vi "GetTemperatureSD.vi"(4 "error in (no error)":errorcluster) -> (0 "error out":errorcluster, 1 "DLL error code":u32, 2 "status":T1, 3 "temperature":i32)   [LabVIEW 2015]
doc: "This function returns the temperature of the detector to the nearest degree. It also gives the status of cooling process.\n\n<B>Parameter:</B>\ntemperature - temperature of the detector\nstatus - status of cooling process\n\n<B>Error codes:</B>\nDRV_NOT_INITIALIZED - System not initialized.\nDRV_ACQUIRING - Acquisition in progress.\nDRV_ERROR_ACK - Unable to communicate with card.\nDRV_TEMP_OFF - Temperature is OFF.\nDRV_TEMP_STABILIZED - Temperature has stabilized at set point.\nDRV_TEMP_NOT_REACHED - Temperature has not reached set point."
uses:
  Error Code Enum typedef.ctl
  DLL/atmcd32d.dll
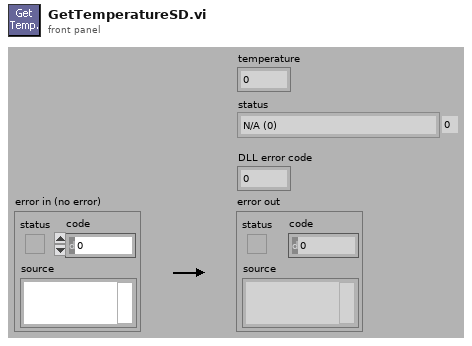
[diagram p1: front panel]
types:
  T1 = typedef "Error Code Enum typedef.ctl" = enum32{"N/A (0)", "DRV_ERROR_CODES", "DRV_SUCCESS", "DRV_VXDNOTINSTALLED", "DRV_ERROR_SCAN", "DRV_ERROR_CHECK_SUM", "DRV_ERROR_FILELOAD", "DRV_UNKNOWN_FUNC", "DRV_ERROR_VXD_INIT", "DRV_ERROR_ADDRESS", "DRV_ERROR_PAGELOCK", "DRV_ERROR_PAGEUNLOCK", "DRV_ERROR_BOARDTEST", "DRV_ERROR_ACK", "DRV_ERROR_UP_FIFO", "DRV_ERROR_PATTERN", "N/A (16)", "DRV_ACQUISITION_ERRORS", "DRV_ACQ_BUFFER", "DRV_ACQ_DOWNFIFO_FULL", "DRV_PROC_UNKONWN_INSTRUCTION", "DRV_ILLEGAL_OP_CODE", "DRV_KINETIC_TIME_NOT_MET", "DRV_ACCUM_TIME_NOT_MET", "DRV_NO_NEW_DATA", "N/A (25)", "DRV_SPOOLERROR", "N/A (27)", "N/A (28)", "N/A (29)", "N/A (30)", "N/A (31)", "N/A (32)", "DRV_TEMPERATURE_CODES", "DRV_TEMPERATURE_OFF", "DRV_TEMPERATURE_NOT_STABILIZED", "DRV_TEMPERATURE_STABILIZED", "DRV_TEMPERATURE_NOT_REACHED", "DRV_TEMPERATURE_OUT_RANGE", "DRV_TEMPERATURE_NOT_SUPPORTED", "DRV_TEMPERATURE_DRIFT", "N/A (41)", "N/A (42)", "N/A (43)", "N/A (44)", "N/A (45)", "N/A (46)", "N/A (47)", "N/A (48)", "DRV_GENERAL_ERRORS", "DRV_INVALID_AUX", "DRV_COF_NOTLOADED", "DRV_FPGAPROG", "DRV_FLEXERROR", "DRV_GPIBERROR", "N/A (55)", "N/A (56)", "N/A (57)", "N/A (58)", "N/A (59)", "N/A (60)", "N/A (61)", "N/A (62)", "N/A (63)", "DRV_DATATYPE", "DRV_DRIVER_ERRORS", "DRV_P1INVALID", "DRV_P2INVALID", "DRV_P3INVALID", "DRV_P4INVALID", "DRV_INIERROR", "DRV_COFERROR", "DRV_ACQUIRING", "DRV_IDLE", "DRV_TEMPCYCLE", "DRV_NOT_INITIALIZED", "DRV_P5INVALID", "DRV_P6INVALID", "DRV_INVALID_MODE", "DRV_INVALID_FILTER", "DRV_I2CERRORS", "DRV_I2CDEVNOTFOUND", "DRV_I2CTIMEOUT", "DRV_P7INVALID", "N/A (84)", "N/A (85)", "N/A (86)", "N/A (87)", "N/A (88)", "N/A (89)", "DRV_IOCERROR", "DRV_VRMVERSIONERROR"}
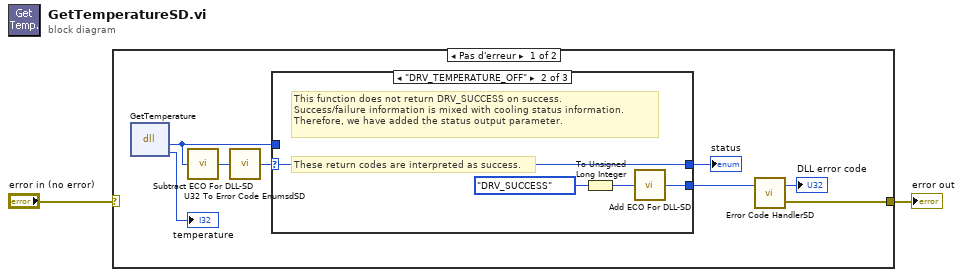
[diagram p0: block diagram]
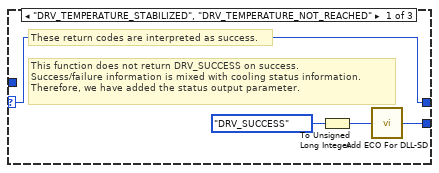
[diagram p2: hidden frame]
diagram:
  n1 = case shown="Pas d'erreur" "error in (no error)" {
    selector: "error in (no error)" -> [_ w21]
    tunnel: [w10 w21] -> w1
    frame No Error {
      n2 = dll-call lib="G:/SD/TRANCON-2015/DLL/Atmcd32d.dll" fn="GetTemperature"() -> (w3:u32, "temperature"=→"temperature":i32)  [unwired: 4 in, 2 out]
      n3 = call "Subtract ECO For DLL-SD.vi"("x"=w3) -> ("x - ECO4DLL"=w7:u32)
      n4 = call "U32 To Error Code EnumsdSD.vi"("U32"=w7) -> ("error code enum"=w6:T1)
      n5 = case shown="\"DRV_TEMPERATURE_OFF\"" w6 {
        selector: w6 -> [w14 w18 w19]
        tunnel: [w14 w18 w19] -> w5
        tunnel: w3 -> [_ _ w20]
        tunnel: [w11 w15 w20] -> w4
        frame "DRV_TEMPERATURE_STABILIZED", "DRV_TEMPERATURE_NOT_REACHED" {
          # "These return codes are interpreted as success."
          # "This function does not return DRV_SUCCESS on success.\nSuccess/failure information is mixed with cooling status information.\nTherefore, we have added the status output parameter."
          n6 = To Unsigned Long Integer(number=Error_Code_Enum_typedef."DRV_SUCCESS" ("error code enum")) -> (unsigned 32bit integer=w12:u32)
          n7 = call "Add ECO For DLL-SD.vi"("x"=w12) -> ("x + ECO4DLL"=w11:u32)
        }
        frame "DRV_TEMPERATURE_OFF" {
          # "These return codes are interpreted as success."
          # "This function does not return DRV_SUCCESS on success.\nSuccess/failure information is mixed with cooling status information.\nTherefore, we have added the status output parameter."
          n8 = To Unsigned Long Integer(number=Error_Code_Enum_typedef."DRV_SUCCESS" ("error code enum")) -> (unsigned 32bit integer=w16:u32)
          n9 = call "Add ECO For DLL-SD.vi"("x"=w16) -> ("x + ECO4DLL"=w15:u32)
        }
        frame Default {
          # "These return codes are interpreted as errors."
        }
      }
      "status" <- w5
      n10 = call "Error Code HandlerSD.vi"("DLL error code"=w4) -> ("error out"=w10:errorcluster, "dup DLL error code"=→"DLL error code":u32)  [unwired: 1 in]
    }
    frame Error {
    }
  }
  "error out" <- w1
